vi "API ID.vi"(11 "API in":refnum<class "API.lvclass">) -> (2 "ID":string)   [LabVIEW 2020, in "Volatus.lvlib" / "API.lvclass"]
uses:
  API.lvclass
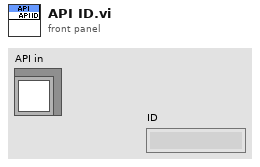
[diagram p1: front panel]
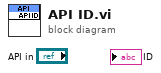
[diagram p0: block diagram]
diagram:
